vi "Read Map Attributes.vi"(8 "error in":errorcluster, 10 "Tree Map In (empty)":T1) -> (0 "error out":errorcluster, 3 "Project out":refnum<class "Project.lvclass">)   [LabVIEW 2019, in "Panther Dashboard.lvlib" / "Project.lvclass"]
uses:
  Project.lvclass
  <vilib>/National Instruments/Tree Map/Tree Map Data.ctl
  Panther Dashboard/Map Attribute--enum.ctl
  Project.lvclass/Project.ctl
  Panther Dashboard/Module type--enum.ctl
  Library/Library.lvclass
  Library/Library.lvclass/Library.ctl
  Write Project Path.vi
  Write Target Name.vi
  Read Libraries.vi
  Library/Write Library Path.vi
  Library/Write Type.vi
  Library/Write Library Description.vi
  Library/Write Dependency.vi
  Write Libraries.vi
  Library/Read Library Path.vi
  Library/Write Library Ref.vi
  Read Project Path.vi
  Read Target Name.vi
  Read Target App Ins Ref.vi
  Panther Dashboard/Panther Dashboard--global.vi
  Panther Dashboard/Panther Dashboard.lvlib
  <vilib>/National Instruments/Tree Map/Tree Map.lvlib
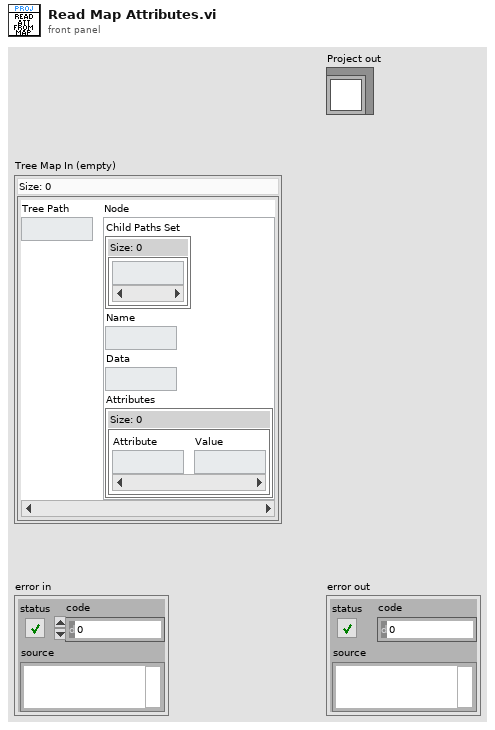
[diagram p1: front panel]
types:
  T1 = typedef "Tree Map.lvlib/Tree Map Data.ctl" = map{string, cluster{"Child Paths Set":set{string}, "Name":string, "Data":string, "Attributes":map{string, string}}}
  T2 = typedef "Panther Dashboard.lvlib/Map Attribute--enum.ctl" = enum16{"Path", "ModuleType", "Module Description", "Dependency?", "Target"}
  T3 = typedef "Panther Dashboard.lvlib/Module type--enum.ctl" = enum16{"Singleton", "Cloneable"}
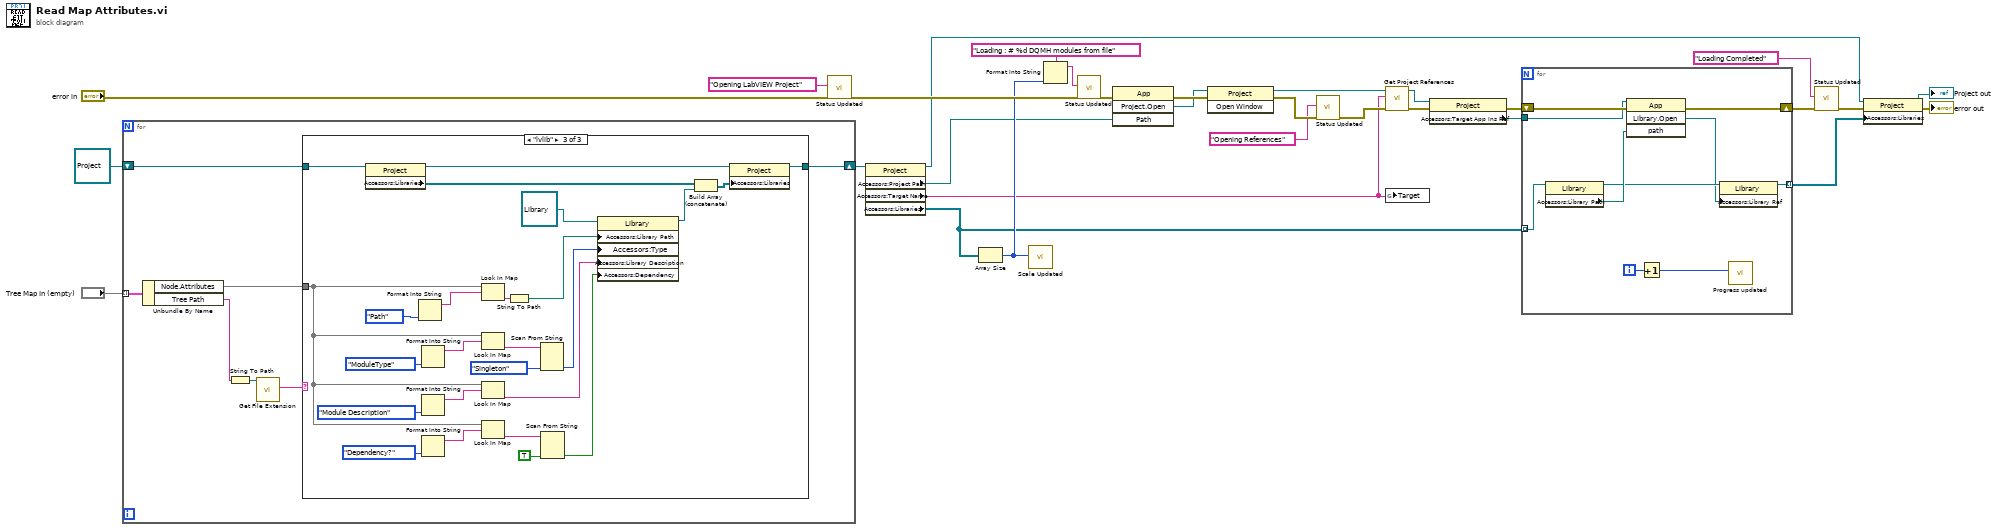
[diagram p0: block diagram]
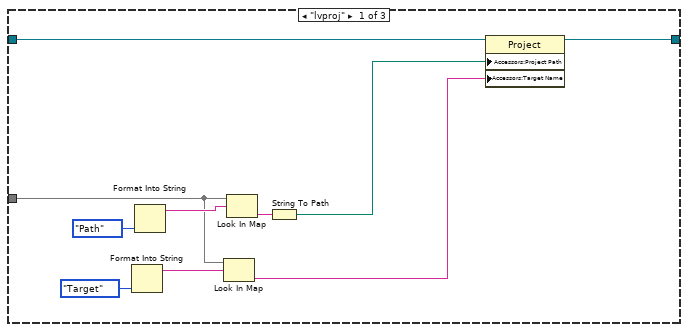
[diagram p2: hidden frame]
diagram:
  n1 = for {
    tunnel: "Tree Map In (empty)" -> [w37] mode=indexing
    shift-right: [w31] -> w9
    shift-left: refnum<class "Project.lvclass"> refnum ("Project In") -> [w32]
    n2 = Unbundle By Name(w37) -> ("Node.Attributes"=w36:map{string, string}, "Tree Path"=w34:string)
    n3 = String To Path(string=w34) -> (path=w35:path)
    n4 = call <vilib>:"Get File Extension.vi"("file"=w35) -> ("lowercase file extension"=w33:string)  [unwired: 6 in, 4 out]
    n5 = case shown="\"lvlib\"" w33 {
      tunnel: w36 -> [w42 _ w65]
      tunnel: w32 -> [w41 w48 w59]
      tunnel: [w40 w48 w57] -> w31
      frame "lvproj" {
        n6 = Format Into String(Map_Attribute--enum."Target" ("Map Attribute")) -> (resulting string=w44:string)  [unwired: 3 in, 1 out]
        n7 = Format Into String(Map_Attribute--enum."Path" ("Map Attribute")) -> (resulting string=w46:string)  [unwired: 3 in, 1 out]
        n8 = Look In Map(map=w42, key=w44) -> (value=w39:string)  [unwired: 1 in, 1 out]
        n9 = Look In Map(map=w42, key=w46) -> (value=w45:string)  [unwired: 1 in, 1 out]
        n10 = String To Path(string=w45) -> (path=w38:path)
        n11 = property class="Project"(reference=w41, "Accessors:Project Path"=w38, "Accessors:Target Name"=w39) -> (reference out=w40:refnum<class "Project.lvclass">)  [unwired: 1 in, 1 out]
      }
      frame Default {
      }
      frame "lvlib" {
        n12 = property class="Project"(reference=w59) -> (reference out=w58:refnum<class "Project.lvclass">, "Accessors:Libraries"=w56:refnum<class "Library.lvclass">[])  [unwired: 1 in, 1 out]
        n13 = Format Into String(Map_Attribute--enum."Path" ("Map Attribute")) -> (resulting string=w72:string)  [unwired: 3 in, 1 out]
        n14 = Format Into String(Map_Attribute--enum."ModuleType" ("Map Attribute")) -> (resulting string=w70:string)  [unwired: 3 in, 1 out]
        n15 = Format Into String(Map_Attribute--enum."Module Description" ("Map Attribute")) -> (resulting string=w67:string)  [unwired: 3 in, 1 out]
        n16 = Format Into String(Map_Attribute--enum."Dependency?" ("Map Attribute")) -> (resulting string=w66:string)  [unwired: 3 in, 1 out]
        n17 = Look In Map(map=w65, key=w72) -> (value=w71:string)  [unwired: 1 in, 1 out]
        n18 = Look In Map(map=w65, key=w70) -> (value=w69:string)  [unwired: 1 in, 1 out]
        n19 = Look In Map(map=w65, key=w67) -> (value=w50:string)  [unwired: 1 in, 1 out]
        n20 = Look In Map(map=w65, key=w66) -> (value=w63:string)  [unwired: 1 in, 1 out]
        n21 = String To Path(string=w71) -> (path=w52:path)
        n22 = Scan From String(input string=w69, default 1=Module_type--enum."Singleton" ("Modules Types Out")) -> (output 1=w51:T3)  [unwired: 3 in, 3 out]
        n23 = Scan From String(input string=w63, default 1=TRUE) -> (output 1=w49:bool)  [unwired: 3 in, 3 out]
        n24 = property class="Library"(reference=refnum<class "Library.lvclass"> refnum ("array"), "Accessors:Library Path"=w52, "Accessors:Type"=w51, "Accessors:Library Description"=w50, "Accessors:Dependency"=w49) -> (reference out=w53:refnum<class "Library.lvclass">)  [unwired: 1 in, 1 out]
        n25 = Build Array (concatenate)(w56, w53) -> (w55:refnum<class "Library.lvclass">[])
        n26 = property class="Project"(reference=w58, "Accessors:Libraries"=w55) -> (reference out=w57:refnum<class "Project.lvclass">)  [unwired: 1 in, 1 out]
      }
    }
  }
  n27 = call "Status Updated.vi"("error in (no error)"="error in", "Status"="Opening LabVIEW Project") -> ("error out"=w25:errorcluster)  [unwired: 9 in]
  n28 = property class="Project"(reference=w9) -> (reference out=w3:refnum<class "Project.lvclass">, "Accessors:Project Path"=w4:path, "Accessors:Target Name"=w5:string, "Accessors:Libraries"=w8:refnum<class "Library.lvclass">[])  [unwired: 1 in, 1 out]
  n29 = Array Size(array=w8) -> (size(s)=w12:i32)
  n30 = call "Scale Updated.vi"("Scale Max"=w12) -> ()  [unwired: 10 in, 1 out]
  n31 = Format Into String(format string="Loading : # %d DQMH modules from file", w12) -> (resulting string=w14:string)  [unwired: 2 in, 1 out]
  n32 = call "Status Updated.vi"("error in (no error)"=w25, "Status"=w14) -> ("error out"=w24:errorcluster)  [unwired: 9 in]
  n33 = invoke class="App" method="Project.Open"(error in=w24, "Path"=w4) -> (error out=w29:errorcluster, "Project:Open"=w17:refnum<vi>)  [unwired: 2 in, 2 out]
  n34 = invoke class="Project" method="Open Window"(reference=w17, error in=w29) -> (reference out=w18:refnum<vi>, error out=w28:errorcluster)  [unwired: 1 in, 1 out]
  n35 = call "Status Updated.vi"("error in (no error)"=w28, "Status"="Opening References") -> ("error out"=w26:errorcluster)  [unwired: 9 in]
  n36 = call "Get Project References.vi"("error in"=w26, "Target Selection"=w5, "Project in"=w18) -> ("error out"=w22:errorcluster, "Project"=w7:refnum<class "Project.lvclass">)  [unwired: 7 in]
  n37 = global write "Panther Dashboard--global.vi" "Target"(w5) -> ()
  n38 = property class="Project"(reference=w7, error in=w22) -> (error out=w21:errorcluster, "Accessors:Target App Ins Ref"=w6:refnum<vi>)  [unwired: 1 out]
  n39 = for {
    shift-right: [w82] -> w30
    shift-left: w21 -> [w83]
    tunnel: w6 -> [w77]
    tunnel: w8 -> [w79] mode=indexing
    tunnel: [w75] -> w2 mode=indexing
    i -> [w81]
    n40 = property class="Library"(reference=w79) -> (reference out=w76:refnum<class "Library.lvclass">, "Accessors:Library Path"=w78:path)  [unwired: 1 in, 1 out]
    n41 = invoke class="App" method="Library.Open"(reference=w77, error in=w83, "path"=w78) -> (error out=w82:errorcluster, "Open Library"=w74:refnum<vi>)  [unwired: 1 in, 2 out]
    n42 = Increment(x=w81) -> (x+1=w80:i32)
    n43 = property class="Library"(reference=w76, "Accessors:Library Ref"=w74) -> (reference out=w75:refnum<class "Library.lvclass">)  [unwired: 1 in, 1 out]
    n44 = call "Progress updated.vi"("Progress"=w80) -> ()  [unwired: 10 in, 1 out]
  }
  n45 = call "Status Updated.vi"("error in (no error)"=w30, "Status"="Loading Completed") -> ("error out"=w23:errorcluster)  [unwired: 9 in]
  n46 = property class="Project"(reference=w3, error in=w23, "Accessors:Libraries"=w2) -> (reference out=→"Project out":refnum<class "Project.lvclass">, error out=→"error out":errorcluster)
